vi "CRC_add.vi"(8 "error in (no error)":errorcluster, 11 "ISO 14443 B UP in":refnum<class "ISO 14443 B UP.lvclass">) -> (0 "error out":errorcluster, 3 "ISO 14443 B UP out":refnum<class "ISO 14443 B UP.lvclass">)   [LabVIEW 2019, in "ISO 14443 B UP.lvclass"]
uses:
  ISO 14443 B UP.lvclass
  TypeDef/Store.ctl
  ISO 14443 B UP.lvclass/ISO 14443 B UP.ctl
  Libraries/CRC/CRC16CITT_B_15.vi
  RFID system.lvclass
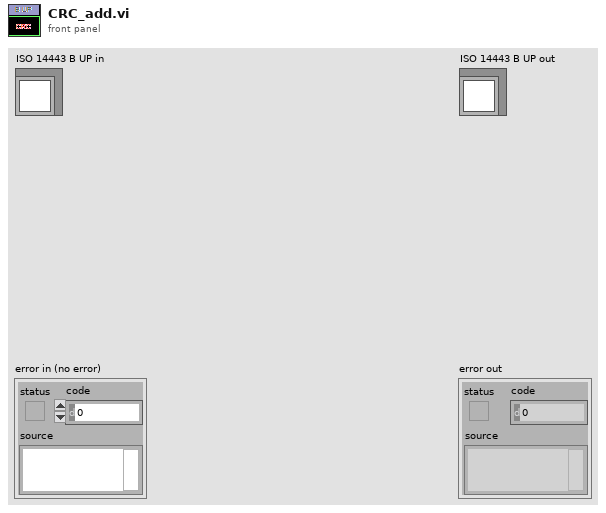
[diagram p1: front panel]
types:
  T1 = typedef "Store.ctl" = enum16{"envelope", "noise", "demSubCar", "CH_frame", "Decode", "demodulate", "in", "out", "sum", "subCarrier", "frame", "command", "encode", "modulate", "encode_UP", "modulate_up", "demod_up", "envelop_up", "sum_up", "out_up", "in_up"}
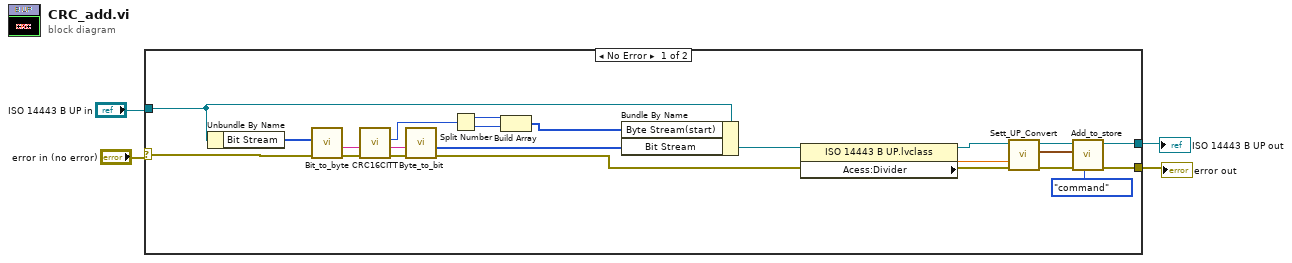
[diagram p0: block diagram]
diagram:
  n1 = case shown="No Error" "error in (no error)" {
    selector: "error in (no error)" -> [w26 w28]
    tunnel: [w20 w28] -> w1
    tunnel: "ISO 14443 B UP in" -> [w25 w27]
    tunnel: [w17 w27] -> w2
    frame No Error {
      n2 = Unbundle By Name(w25) -> ("Bit Stream"=w24:u8[])
      n3 = call "Bit_to_byte.vi"("Error In"=w26, "Array of bit"=w24) -> ("Error Out"=w13:errorcluster, "BYTE"=w14:string)  [unwired: 7 in, 1 out]
      n4 = call-poly "CRC16CITT.vi"("Error In"=w13, "DATA PACKET"=w14) -> ("Error Out"=w12:errorcluster, "DATA PACKET+CRC"=w11:string, "CRC out"=w8:u16)  [unwired: 7 in]
      n5 = call "Byte_to_bit.vi"("Error In"=w12, "BYTE"=w11) -> ("Error Out"=w22:errorcluster, "Arrray of bit (str)"=w23:u8[])  [unwired: 5 in, 1 out]
      n6 = Split Number(x=w8) -> (hi(x)=w7:u8, lo(x)=w6:u8)
      n7 = Build Array(w7, w6) -> (w5:u8[])
      n8 = Bundle By Name(cluster=w25, "Byte Stream(start)"=w5, "Bit Stream"=w23) -> (w19:refnum<class "ISO 14443 B UP.lvclass">)
      n9 = property class="ISO 14443 B UP.lvclass"(reference=w19) -> (reference out=w10:refnum<class "ISO 14443 B UP.lvclass">, "Acess:Divider"=w9:dbl)  [unwired: 1 in, 1 out]
      n10 = call-dynamic "Sett_UP_Convert.vi"("error in (no error)"=w22, "Divider(1)"=w9, "ISO 14443 B UP in"=w10) -> ("error out"=w21:errorcluster, "Waveform"=w15:waveform(dbl), "ISO 14443 B UP out"=w18:refnum<class "ISO 14443 B UP.lvclass">)  [unwired: 6 in]
      n11 = call "Add_to_store.vi"("Store"=Store."command", "error in (no error)"=w21, "Waveform"=w15, "RFID system in"=w18) -> ("error out"=w20:errorcluster, "RFID system out"=w17:refnum<class "ISO 14443 B UP.lvclass">)  [unwired: 6 in]
    }
    frame Error {
    }
  }
  "error out" <- w1
  "ISO 14443 B UP out" <- w2
